vi "和校验-16.vi"(8 "错误输入":errorcluster caption="错误输入（无错误）", 11 "需校验字符串":string) -> (0 "错误输出":errorcluster, 3 "校验":string)   [LabVIEW 2014, in "校验.lvlib"]
doc: "<B>输入端子 需校验字符串 ：</B>输入需要校验的字符串\n<B>输出端子 校验：</B>将需要校验的字符串，通过校验和-16算法，求出校验\n\n公式：将字符串两两拆分，然后相加，最后除以65536.\n编写人：曾嘉康\n编写时间：2014/12/18"
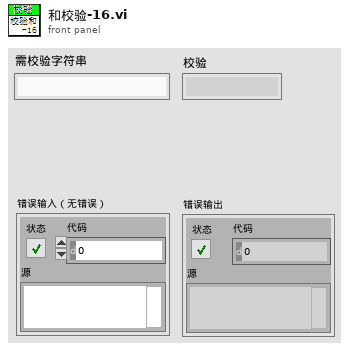
[diagram p1: front panel]
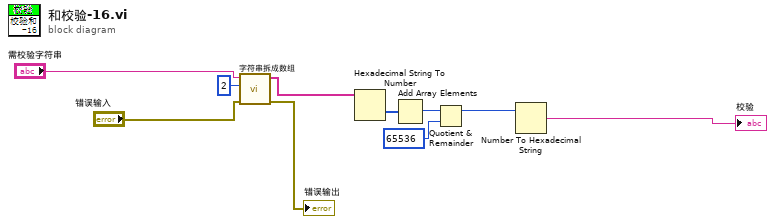
[diagram p0: block diagram]
diagram:
  n1 = call "字符串拆成数组.vi"("错误输入"="错误输入", "索引"=2, "字符串"="需校验字符串") -> ("错误输出"=→"错误输出":errorcluster, "数组"=w2:string[])  [unwired: 7 in]
  n2 = Hexadecimal String To Number(string=w2) -> (number=w7:u32[])  [unwired: 2 in, 1 out]
  n3 = Add Array Elements(numeric array=w7) -> (sum=w6:u32)
  n4 = Quotient & Remainder(x=w6, y=u32 65536) -> (x-y*floor(x/y)=w3:u32)  [unwired: 1 out]
  n5 = Number To Hexadecimal String(2:w3) -> (0:→"校验":string)  [unwired: 1 in]
